vi "Sub_Set_Output_Switch.vi"(2 "error in":errorcluster, 3 "Enabled? (False)":bool, 4 "i":i32, 5 "AgB29xxLib.IAgB29xx2":refnum<k7>) -> (0 "error out":errorcluster, 1 "AgB29xxLib.IAgB29xx2 2":refnum<k7>)   [LabVIEW 2009]
panel:
  # "Sub VI: Set Output Switch"
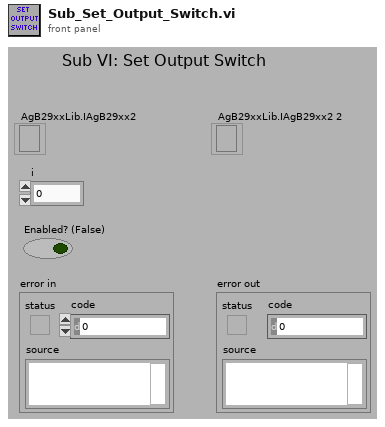
[diagram p1: front panel]
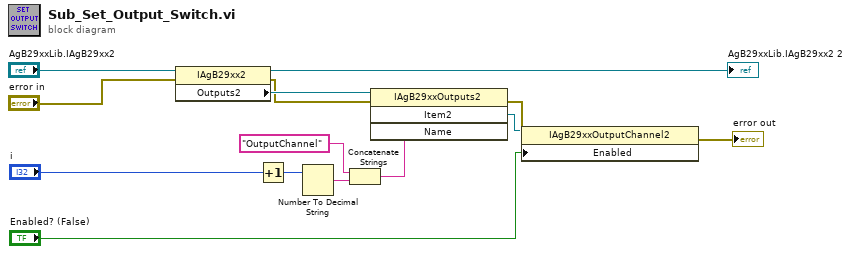
[diagram p0: block diagram]
diagram:
  n1 = property class="IAgB29xx2"(reference="AgB29xxLib.IAgB29xx2", error in="error in") -> (reference out=→"AgB29xxLib.IAgB29xx2 2":refnum<k7>, error out=w10:errorcluster, "Outputs2"=w11:refnum<k7>)
  n2 = Increment(x="i") -> (x+1=w9:i32)
  n3 = Number To Decimal String(number=w9) -> (decimal integer string=w8:string)  [unwired: 1 in]
  n4 = Concatenate Strings("OutputChannel" ("string"), w8) -> (w6:string)
  n5 = invoke class="IAgB29xxOutputs2" method="Item2"(reference=w11, error in=w10, "Name"=w6) -> (error out=w4:errorcluster, "Item2"=w3:refnum<k7>)  [unwired: 1 in, 2 out]
  n6 = property class="IAgB29xxOutputChannel2"(reference=w3, error in=w4, "Enabled"="Enabled? (False)") -> (error out=→"error out":errorcluster)  [unwired: 1 out]
